vi "Measure Cap.vi"(7 "Measurement Id":string="CFree", 8 "error in (no error)":errorcluster, 9 "VNAs Measurement Parameters":T2, 10 "Pins":string[](array[string])=["RF"], 11 "Semiconductor Module Context":T1) -> (0 "error out":errorcluster, 2 "Multisite Cap Data":dbl[][](array[numeric]), 3 "Semiconductor Module Context Out":T1)   [LabVIEW 2013]
uses:
  <vilib>/NI_TestStand_SemiconductorModule/NI_TestStand_Semiconductor_Module.lvlibp/PinMap/General/SemiconductorModuleContext.ctl
  VNAs Measurement Parameters.ctl
  <vilib>/NI_TestStand_SemiconductorModule/NI_TestStand_Semiconductor_Module.lvlibp/PinMap/General/Publish/PublishDataDouble2D.vi
  Pin Map API/VNA Custom Instrument.lvlib
  <vilib>/NI_TestStand_SemiconductorModule/NI_TestStand_Semiconductor_Module.lvlibp
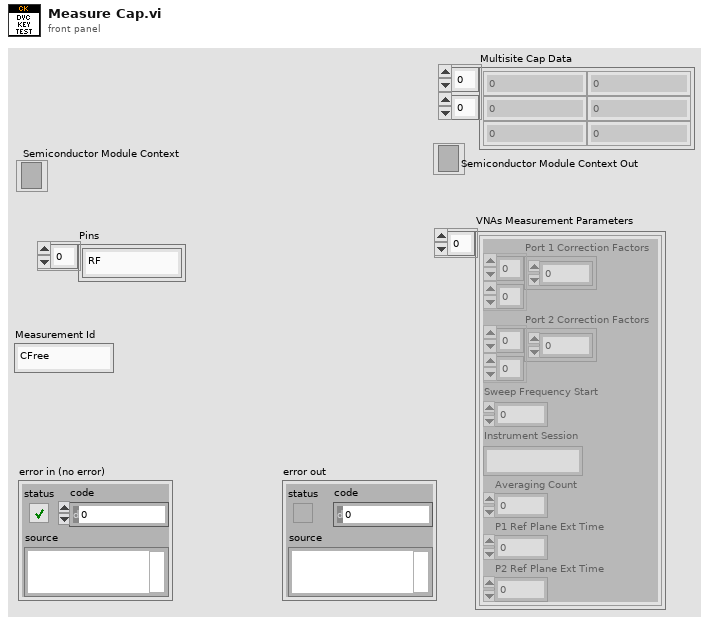
[diagram p1: front panel]
types:
  T1 = typedef "NI_TestStand_Semiconductor_Module.lvlibp/SemiconductorModuleContext.ctl" = refnum<k7>
  T2 = typedef "VNAs Measurement Parameters.ctl" = cluster{"Port 1 Correction Factors":cdb[][], "Port 2 Correction Factors":cdb[][], "Sweep Frequency Start":dbl, "Instrument Session":string, "Averaging Count":i32, "P1 Ref Plane Ext Time":dbl, "P2 Ref Plane Ext Time":dbl}[]
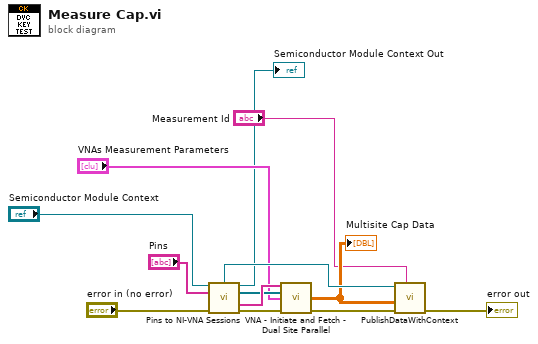
[diagram p0: block diagram]
diagram:
  n1 = call "Pins to NI-VNA Sessions.vi"("Semiconductor Module Context"="Semiconductor Module Context", "Pins"="Pins", "error in (no error)"="error in (no error)") -> ("Pin Query Context"=w12:refnum<class "MultiplePinMultipleSessionQueryContext.lvclass">, "Semiconductor Module Context Out"=→"Semiconductor Module Context Out":T1, "Instrument Sessions"=w9:refnum<k15>[], "Channel Lists"=w10:string[], "error out"=w11:errorcluster)  [unwired: 8 in]
  n2 = call "VNA - Initiate and Fetch - Dual Site Parallel.vi"("Channel Lists In"=w10, "Instrument Sessions In"=w9, "VNAs Measurement Parameters"="VNAs Measurement Parameters", "error in (no error)"=w11) -> ("Multisite Cap Data"=w4:dbl[][], "error out"=w2:errorcluster)  [unwired: 6 in, 4 out]
  "Multisite Cap Data" <- w4
  n3 = call-poly <vilib>:"PublishDataWithContext.vi"("Published Data Id"="Measurement Id", "error in (no error)"=w2, "Data In"=w4, "Pin Query Context"=w12) -> ("error out"=→"error out":errorcluster)  [unwired: 6 in, 1 out]
